vi "FTW-CodeGen-GenerateCode.vi"(0 "State In":T2 {"Actor Interface"."Bounds"."Left" format="%dpx"; "Actor Interface"."Bounds"."Top" format="%dpx"; "Actor Interface"."Bounds"."Right" format="%dpx"; "Actor Interface"."Bounds"."Bottom" format="%dpx"}, 5 "XRef":refnum<vi>, 7 "Terms":T1(array[cluster]), 9 "Diagram":refnum<vi>) -> (4 "State Out":T2 {"Actor Interface"."Bounds"."Left" format="%dpx"; "Actor Interface"."Bounds"."Top" format="%dpx"; "Actor Interface"."Bounds"."Right" format="%dpx"; "Actor Interface"."Bounds"."Bottom" format="%dpx"}, 6 "Reply":string[](array[string]), 8 "Generated Code?":bool)   [LabVIEW 2015, in "FTW-Actor-Spawn.xnode"]
uses:
  FTW-Actor-Spawn.xnode
  FTW-CodeGen-State.ctl
  FTW-CodeGen-XNodeReplyType.ctl
panel:
  # "Inputs"
  # "Outputs"
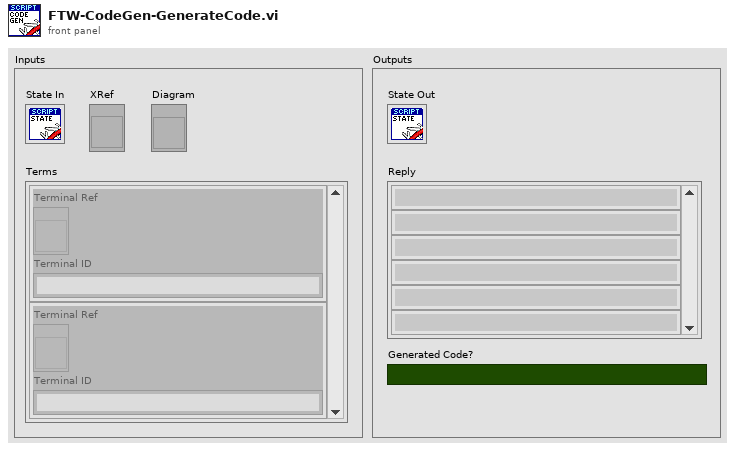
[diagram p1: front panel]
types:
  T1 = cluster{"Terminal Ref":refnum<vi>, "Terminal ID":string}[]
  T2 = typedef "FTW-Actor-Spawn.xnode/FTW-CodeGen-State.ctl" = cluster{"Path Wired?":bool, "Actor Interface":cluster{"Name":string, "Type":variant, "Bounds":cluster{"Left":i32, "Top":i32, "Right":i32, "Bottom":i32}, "Input":bool, "Recommended":bool, "Required":bool, "Dynamic Dispatch":bool, "On Interface":bool, "\"The\" Config Terminal":bool}[], "Config Terminal Index":i32}
  T3 = typedef "FTW-CodeGen-XNodeReplyType.ctl" = enum16{"UpdateState", "AdaptToInputs", "AdaptAndAugment", "CosmeticUpdate", "NoReply"}
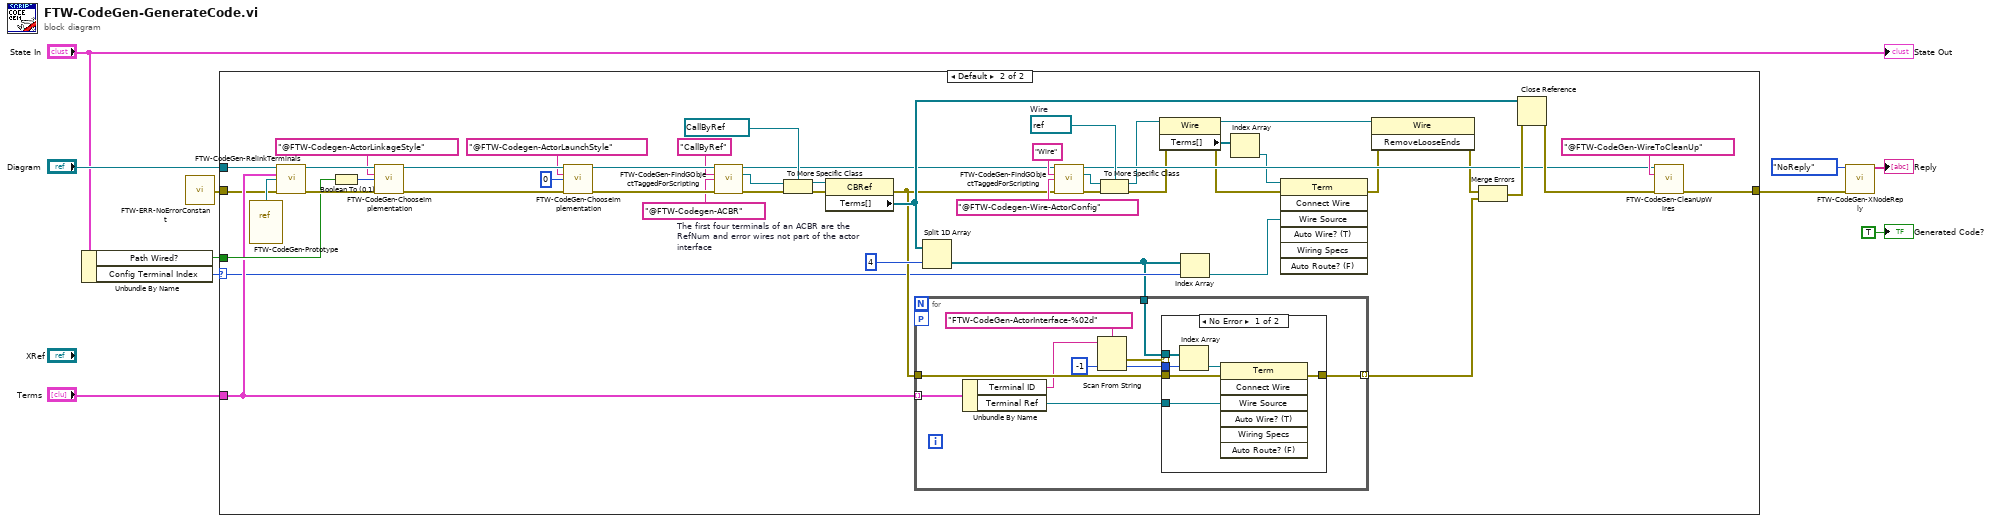
[diagram p0: block diagram]
diagram:
  n1 = Unbundle By Name("State In") -> ("Path Wired?"=w1:bool, "Config Terminal Index"=w3:i32)
  n2 = call "FTW-ERR-NoErrorConstant.vi"() -> ("no error"=w2:errorcluster)
  n3 = case shown="Default" w3 {
    selector: w3 -> [_ w15]
    tunnel: "Diagram" -> [_ w58]
    tunnel: w1 -> [_ w54]
    tunnel: [w11 w47] -> w5
    tunnel: "Terms" -> [_ w38]
    tunnel: w2 -> [w11 w32]
    frame -1 {
    }
    frame Default {
      w27 = refnum<vi> refnum  # Wire
      w36 = 4  # The first four terminals of an ACBR are the RefNum and error wires not part of the actor interface
      n4 = vi-ref "FTW-CodeGen-Prototype.vi"() -> (w59:refnum<vi>)
      n5 = call "FTW-CodeGen-RelinkTerminals.vi"("Diagram"=w58, "Terms"=w38, "PrototypeVI"=w59, "error in"=w32) -> ("Diagram out"=w57:refnum<vi>, "error out"=w56:errorcluster)  [unwired: 10 in]
      n6 = Boolean To (0,1)(Boolean=w54) -> (0, 1=w53:i16)
      n7 = call "FTW-CodeGen-ChooseImplementation.vi"("GObject to Traverse"=w57, "Diagram Disable Structure Label"="@FTW-Codegen-ActorLinkageStyle", "Frame to Keep"=w53, "error in"=w56) -> ("GObject to Traverse out"=w52:refnum<vi>, "error out"=w49:errorcluster)  [unwired: 10 in]
      n8 = call "FTW-CodeGen-ChooseImplementation.vi"("GObject to Traverse"=w52, "Diagram Disable Structure Label"="@FTW-Codegen-ActorLaunchStyle", "Frame to Keep"=u32 0, "error in"=w49) -> ("GObject to Traverse out"=w46:refnum<vi>, "error out"=w45:errorcluster)  [unwired: 10 in]
      n9 = call "FTW-CodeGen-FindGObjectTaggedForScripting.vi"("GObject to Traverse"=w46, "Class Name"="CallByRef", "Label Prefix to uniquely identify node"="@FTW-Codegen-ACBR", "error in"=w45) -> ("GObject to Traverse out"=w26:refnum<vi>, "GObject"=w42:refnum<vi>, "error out"=w40:errorcluster)  [unwired: 9 in]
      n10 = To More Specific Class(target class=refnum<vi> refnum ("GObject"), reference=w42, error in=w40) -> (specific class reference=w12:refnum<vi>, error out=w39:errorcluster)
      n11 = property class="CBRef"(reference=w12, error in=w39) -> (error out=w24:errorcluster, "Terms[]"=w33:refnum<vi>[])  [unwired: 1 out]
      n12 = Split 1D Array(array=w33, index=w36) -> (second subarray=w14:refnum<vi>[])  [unwired: 1 out]
      n13 = for {
        tunnel: w14 -> [w64]
        tunnel: w38 -> [w67] mode=indexing
        tunnel: w24 -> [w68]
        tunnel: [w69] -> w37 mode=indexing
        workers-P: _ -> [_]
        n14 = Unbundle By Name(w67) -> ("Terminal ID"=w62:string, "Terminal Ref"=w66:refnum<vi>)
        n15 = Scan From String(format string="FTW-CodeGen-ActorInterface-%02d", input string=w62, default 1=-1 ("default value 1")) -> (error out=w61:errorcluster, output 1=w63:i32)  [unwired: 2 in, 2 out]
        n16 = case shown="No Error" w61 {
          tunnel: [w75 w76] -> w69
          tunnel: w68 -> [w74 w76]
          tunnel: w66 -> [w73 _]
          tunnel: w64 -> [w72 _]
          tunnel: w63 -> [w71 _]
          frame No Error {
            n17 = Index Array(array=w72, index=w71) -> (element=w70:refnum<vi>)
            n18 = invoke class="Term" method="Connect Wire"(reference=w70, error in=w74, "Wire Source"=w73) -> (error out=w75:errorcluster)  [unwired: 4 in, 6 out]
          }
          frame Error {
          }
        }
      }
      n19 = call "FTW-CodeGen-FindGObjectTaggedForScripting.vi"("GObject to Traverse"=w26, "Class Name"="Wire", "Label Prefix to uniquely identify node"="@FTW-Codegen-Wire-ActorConfig", "error in"=w24) -> ("GObject to Traverse out"=w25:refnum<vi>, "GObject"=w29:refnum<vi>, "error out"=w28:errorcluster)  [unwired: 9 in]
      n20 = To More Specific Class(target class=w27, reference=w29, error in=w28) -> (specific class reference=w23:refnum<vi>, error out=w20:errorcluster)
      n21 = property class="Wire"(reference=w23, error in=w20) -> (reference out=w18:refnum<vi>, error out=w19:errorcluster, "Terms[]"=w22:refnum<vi>[])
      n22 = Index Array(array=w14, index=w15) -> (element=w13:refnum<vi>)
      n23 = Index Array(array=w22) -> (element=w21:refnum<vi>)  [unwired: 1 in]
      n24 = invoke class="Term" method="Connect Wire"(reference=w21, error in=w19, "Wire Source"=w13) -> (error out=w17:errorcluster)  [unwired: 4 in, 6 out]
      n25 = invoke class="Wire" method="RemoveLooseEnds"(reference=w18, error in=w17) -> (error out=w16:errorcluster)  [unwired: 1 in, 2 out]
      n26 = Merge Errors(w16, w37) -> (w35:errorcluster)
      n27 = Close Reference(reference=w33, error in (no error)=w35) -> (error out=w34:errorcluster)
      n28 = call "FTW-CodeGen-CleanUpWires.vi"("GObject to Traverse"=w25, "Wire Label Patterns to Clean Up"="@FTW-CodeGen-WireToCleanUp" ("Wire Label"), "error in"=w34) -> ("error out"=w47:errorcluster)  [unwired: 11 in, 1 out]
    }
  }
  n29 = call "FTW-CodeGen-XNodeReply.vi"("XNode Reply Type"=FTW-CodeGen-XNodeReplyType."NoReply", "error in"=w5) -> ("Reply"=→"Reply":string[])  [unwired: 13 in]
  "State Out" <- "State In"
  "Generated Code?" <- TRUE ("Generated Code?")
